vi "Calculate_Gradient.vi"() -> (0 "New Values In":string[][](array[string])=[["Test data5"]], 1 "New Chs In":string[](array[string])=["30-10-03:New:Channel new5"])   [LabVIEW 2021]
uses:
  Results_plotter_Global.vi
  Data plotting/subVIs/Plot_Values_Global.vi
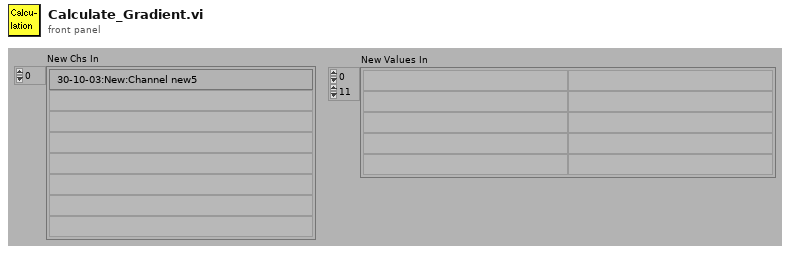
[diagram p1: front panel]
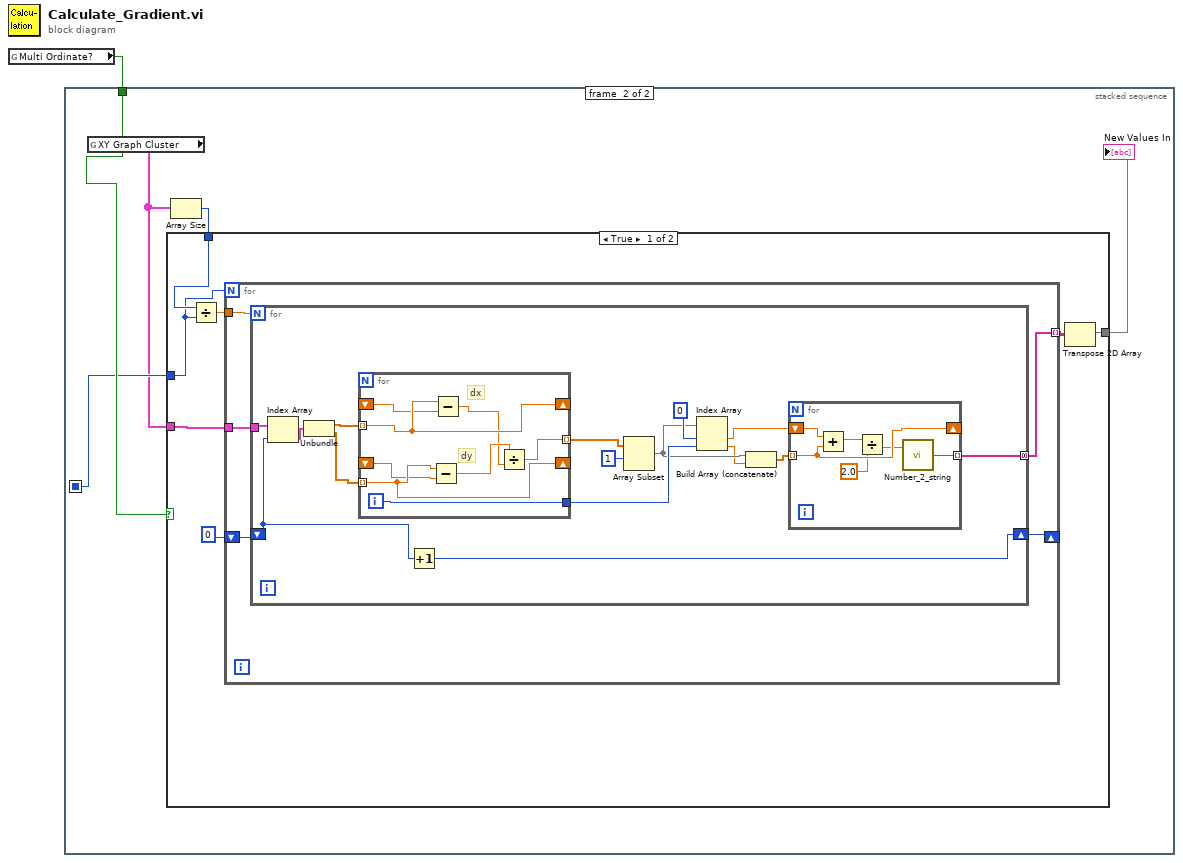
[diagram p0: block diagram]
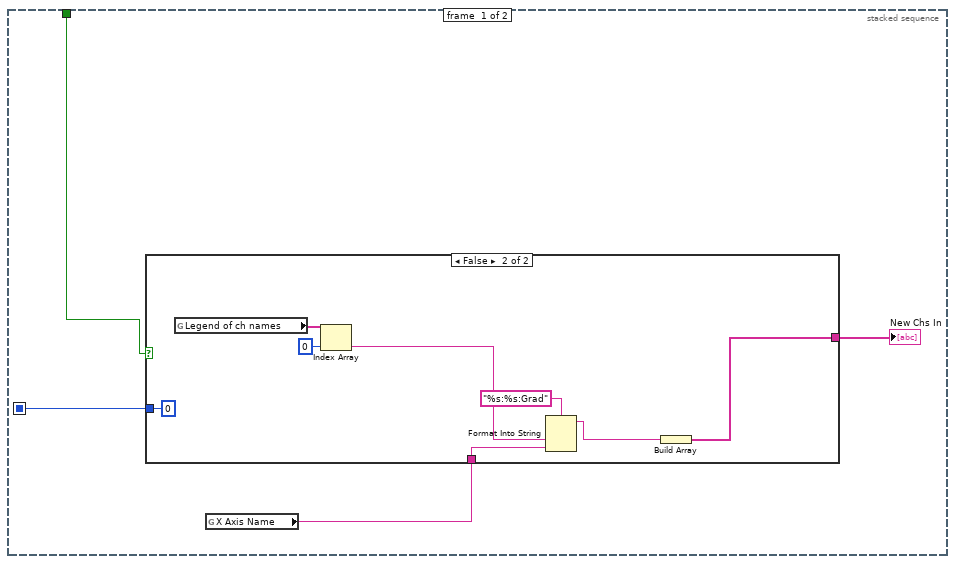
[diagram p2: hidden frame]
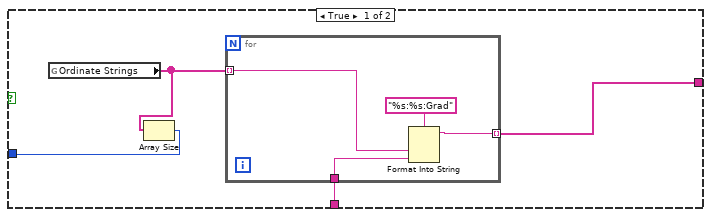
[diagram p3: hidden frame]
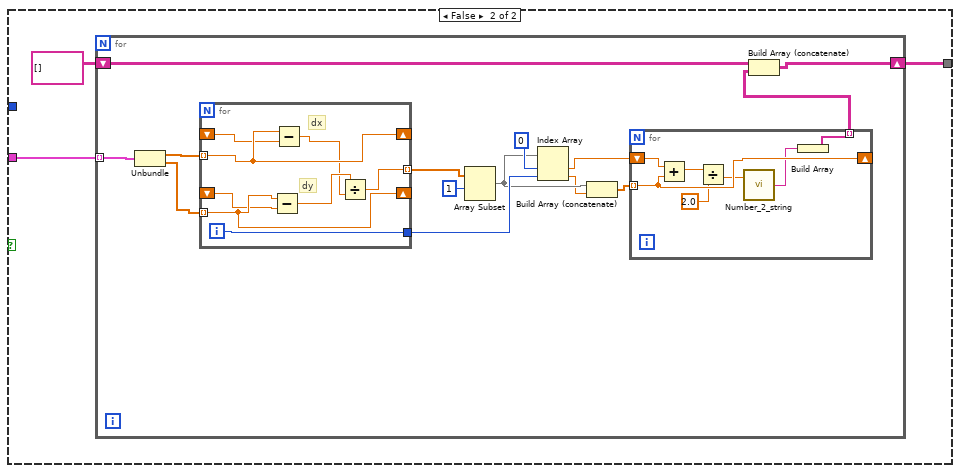
[diagram p4: hidden frame]
diagram:
  n1 = global read "Results_plotter_Global.vi" "Multi Ordinate?"() -> (w1:bool)
  n2 = stacked-sequence {
    seq-local: [w3 _] -> [_ w23]
    tunnel: w1 -> [w2 w25]
    frame #0 {
      n3 = global read "Results_plotter_Global.vi" "X Axis Name"() -> (w4:string)
      n4 = case shown="False" w2 {
        tunnel: [w8 w19] -> w5
        tunnel: w4 -> [w9 w17]
        tunnel: [w6 0] -> w3
        frame True {
          n5 = global read "Results_plotter_Global.vi" "Ordinate Strings"() -> (w7:string[])
          n6 = Array Size(array=w7) -> (size(s)=w6:i32)
          n7 = for {
            tunnel: w9 -> [w13]
            tunnel: w7 -> [w11] mode=indexing
            tunnel: [w10] -> w8 mode=indexing
            n8 = Format Into String(format string="%s:%s:Grad", w11, w13) -> (resulting string=w10:string)  [unwired: 2 in, 1 out]
          }
        }
        frame False {
          n9 = global read "Results_plotter_Global.vi" "Legend of ch names"() -> (w20:string[])
          n10 = Index Array(array=w20, index=0) -> (element=w18:string)
          n11 = Format Into String(format string="%s:%s:Grad", w18, w17) -> (resulting string=w15:string)  [unwired: 2 in, 1 out]
          n12 = Build Array(w15) -> (w19:string[])
        }
      }
      "New Chs In" <- w5
    }
    frame #1 {
      n13 = global read "Plot_Values_Global.vi" "XY Graph Cluster"() -> (w22:cluster{dbl[], dbl[]}[])
      n14 = Array Size(array=w22) -> (size(s)=w24:i32)
      n15 = case shown="True" w25 {
        tunnel: w22 -> [w33 w70]
        tunnel: [w27 w68] -> w26
        tunnel: w24 -> [w32 _]
        tunnel: w23 -> [w29 _]
        frame True {
          n16 = Divide(x=w32, y=w29) -> (x/y=w31:dbl)
          n17 = for {
            N: w29 -> [_]
            tunnel: w33 -> [w38]
            tunnel: w31 -> [w37]
            shift-right: [w35] -> _
            shift-left: 0 -> [w36]
            tunnel: [w34] -> w28 mode=indexing
            n18 = for {
              N: w37 -> [_]
              tunnel: w38 -> [w42]
              tunnel: [w43] -> w34 mode=concatenating
              shift-right: [w40] -> w35
              shift-left: w36 -> [w41]
              n19 = Index Array(array=w42, index=w41) -> (element=w39:cluster{dbl[], dbl[]})
              n20 = Unbundle(w39) -> (w53:dbl[], w52:dbl[])
              n21 = for {
                shift-right: [w67] -> _
                shift-left: _ -> [w66]
                shift-right: [w65] -> _
                shift-left: _ -> [w64]
                tunnel: w53 -> [w67] mode=indexing
                tunnel: w52 -> [w65] mode=indexing
                tunnel: [w61] -> w50 mode=indexing
                tunnel: [w60] -> w48
                i -> [w60]
                # "dy"
                # "dx"
                n22 = Subtract(x=w65, y=w64) -> (x-y=w63:dbl)
                n23 = Subtract(x=w67, y=w66) -> (x-y=w62:dbl)
                n24 = Divide(x=w63, y=w62) -> (x/y=w61:dbl)
              }
              n25 = Increment(x=w41) -> (x+1=w40:i32)
              n26 = Array Subset(array=w50, index=1) -> (w46:dbl[])  [unwired: 1 in]
              n27 = Index Array(array=w46, index #1=0 ("index"), index #2=w48) -> (element #1=w49:dbl, element #2=w45:dbl)
              n28 = Build Array (concatenate)(w46, w45) -> (w44:dbl[])
              n29 = for {
                shift-right: [w58] -> _
                shift-left: w49 -> [w59]
                tunnel: w44 -> [w58] mode=indexing
                tunnel: [w54] -> w43 mode=indexing
                n30 = Add(x=w59, y=w58) -> (x+y=w57:dbl)
                n31 = Divide(x=w57, y=2.0) -> (x/y=w55:dbl)
                n32 = call "Number_2_string.vi"("number"=w55) -> ("String"=w54:string)  [unwired: 1 in]
              }
            }
          }
          n33 = Transpose 2D Array(2D array=w28) -> (transposed array=w27:string[][])
        }
        frame False {
          n34 = for {
            tunnel: w70 -> [w71] mode=indexing
            shift-right: [w83] -> w68
            shift-left: string[][] [] -> [w84]
            n35 = Unbundle(w71) -> (w82:dbl[], w81:dbl[])
            n36 = for {
              shift-right: [w99] -> _
              shift-left: _ -> [w98]
              shift-right: [w97] -> _
              shift-left: _ -> [w96]
              tunnel: w82 -> [w99] mode=indexing
              tunnel: w81 -> [w97] mode=indexing
              tunnel: [w93] -> w79 mode=indexing
              tunnel: [w92] -> w77
              i -> [w92]
              # "dy"
              # "dx"
              n37 = Subtract(x=w97, y=w96) -> (x-y=w95:dbl)
              n38 = Subtract(x=w99, y=w98) -> (x-y=w94:dbl)
              n39 = Divide(x=w95, y=w94) -> (x/y=w93:dbl)
            }
            n40 = Array Subset(array=w79, index=1) -> (w75:dbl[])  [unwired: 1 in]
            n41 = Index Array(array=w75, index #1=0 ("index"), index #2=w77) -> (element #1=w78:dbl, element #2=w74:dbl)
            n42 = Build Array (concatenate)(w75, w74) -> (w73:dbl[])
            n43 = for {
              shift-right: [w90] -> _
              shift-left: w78 -> [w91]
              tunnel: w73 -> [w90] mode=indexing
              tunnel: [w87] -> w72 mode=indexing
              n44 = Add(x=w91, y=w90) -> (x+y=w89:dbl)
              n45 = Divide(x=w89, y=2.0) -> (x/y=w86:dbl)
              n46 = call "Number_2_string.vi"("number"=w86) -> ("String"=w85:string)  [unwired: 1 in]
              n47 = Build Array(w85) -> (w87:string[])
            }
            n48 = Build Array (concatenate)(w84, w72) -> (w83:string[][])
          }
        }
      }
      "New Values In" <- w26
    }
  }
